vi "cameratest.vi"(11 "return value":u8[][][](array[numeric])) -> (3 "Webcam footage":picture)   [LabVIEW 2023]
uses:
  <vilib>/picture/picture.llb/Draw True-Color Pixmap.vi
panel:
  out "Colour":u32[][](array[numeric])
  out "camera open":errorcluster
  out "python version":errorcluster
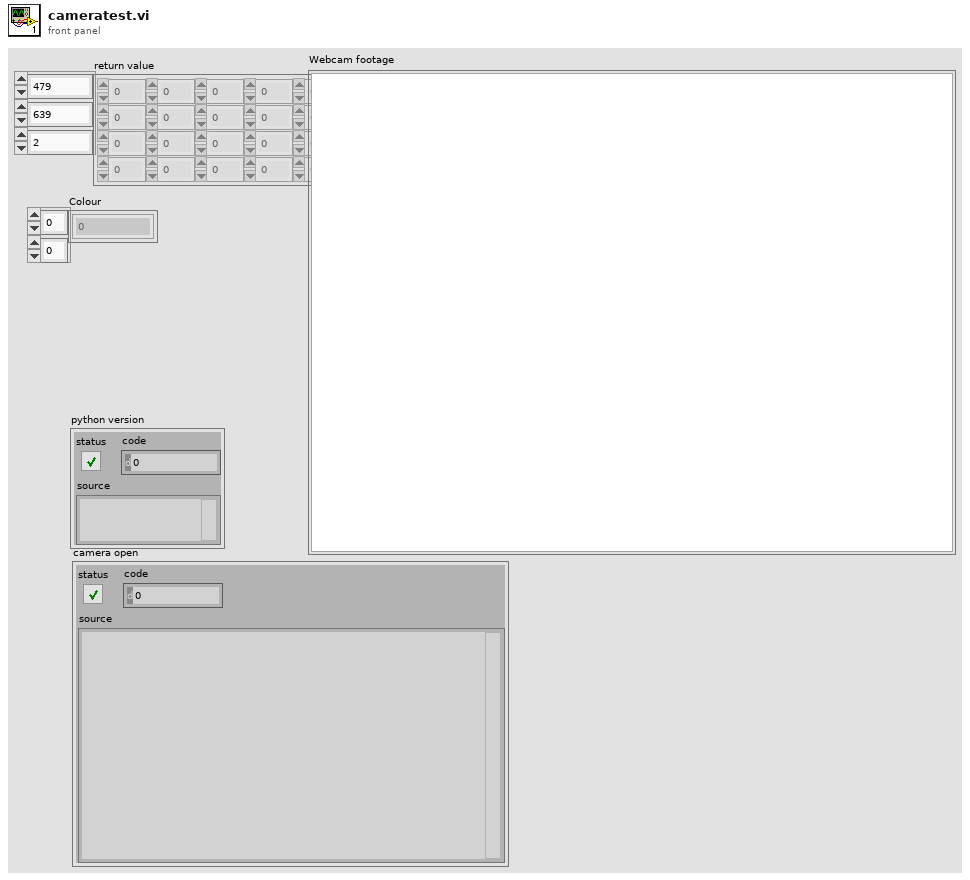
[diagram p1: front panel]
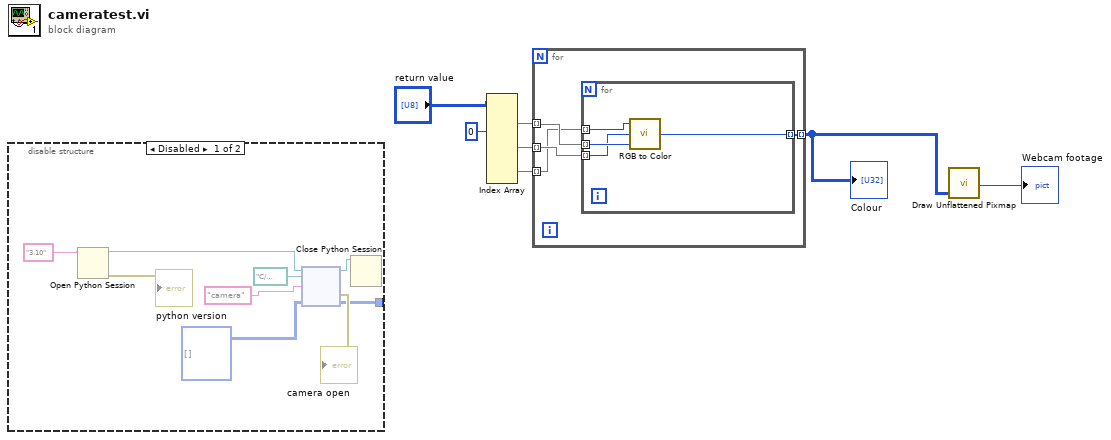
[diagram p0: block diagram]
diagram:
  n1 = disable-structure shown="Disabled" {
    disable-tunnel: [w9 _] -> _
    frame Disabled {
      n2 = Open Python Session(python version="3.10" ("Python version")) -> (session out=w13:refnum<k35>, error out=→"python version":errorcluster)  [unwired: 2 in]
      n3 = node(w13, path "C:/Users/User/source/repos/PythonCameraTest/PythonCameraTest/PythonCameraTest.py" ("module path"), "camera" ("function name"), u8[][][] []) -> (w10:refnum<k35>, →"camera open":errorcluster, w9:u8[][][])  [unwired: 1 in, 2 out]
      n4 = Close Python Session(session in=w10) -> ()  [unwired: 1 in, 1 out]
    }
    frame Enabled {
    }
  }
  n5 = Index Array(array="return value", index (dim 2) #1=0 ("disabled index (col)")) -> (element #1=w6:u8[][], element #2=w5:u8[][], element #3=w4:u8[][])  [unwired: 8 in]
  n6 = for {
    tunnel: w6 -> [w19] mode=indexing
    tunnel: w5 -> [w18] mode=indexing
    tunnel: w4 -> [w17] mode=indexing
    tunnel: [w20] -> w3 mode=indexing
    n7 = for {
      tunnel: [w24] -> w20 mode=indexing
      tunnel: w19 -> [w23] mode=indexing
      tunnel: w18 -> [w22] mode=indexing
      tunnel: w17 -> [w21] mode=indexing
      n8 = call <vilib>:"RGB to Color.vi"("B"=w23, "G"=w22, "R"=w21) -> ("Color"=w24:u32)
    }
  }
  "Colour" <- w3
  n9 = call-poly <vilib>:"Draw Unflattened Pixmap.vi"("data (RGB format)"=w3) -> ("new picture"=→"Webcam footage":picture)  [unwired: 8 in]
